vi "TPI RF on off.vi"(8 "Error in (no error)":errorcluster, 9 "RF on?":bool, 11 "VISA resource name":refnum<visa-resource-name>) -> (0 "Error out":errorcluster, 3 "VISA resource name out":refnum<visa-resource-name>)   [LabVIEW 2019]
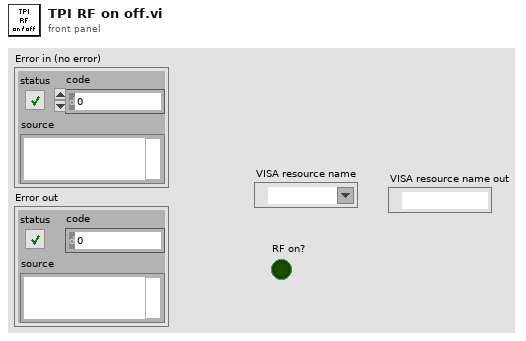
[diagram p1: front panel]
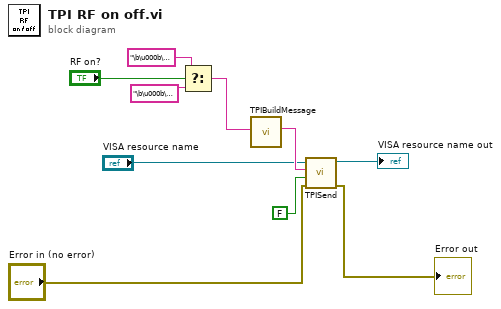
[diagram p0: block diagram]
diagram:
  n1 = Select(t="\b\u000b\u0001" ("Command"), s="RF on?", f="\b\u000b\u0000" ("Command")) -> (s? t:f=w3:string)
  n2 = call "TPIBuildMessage.vi"("Command"=w3) -> ("Message"=w9:string)  [unwired: 10 in]
  n3 = call "TPISend.vi"("error in (no error)"="Error in (no error)", "Read Responce"=FALSE, "write buffer"=w9, "VISA resource name"="VISA resource name") -> ("error out"=→"Error out":errorcluster, "VISA resource name out"=→"VISA resource name out":refnum<visa-resource-name>)  [unwired: 5 in, 1 out]
